vi "Prechirper response process.vi"(8 "error in (no error)":errorcluster, 10 "Prechirper response":string, 11 "Pre-chirper commands":T1) -> (0 "error out":errorcluster, 2 "offset past number":i32, 3 "number":dbl)   [LabVIEW 2020]
uses:
  Prechirper commands.ctl
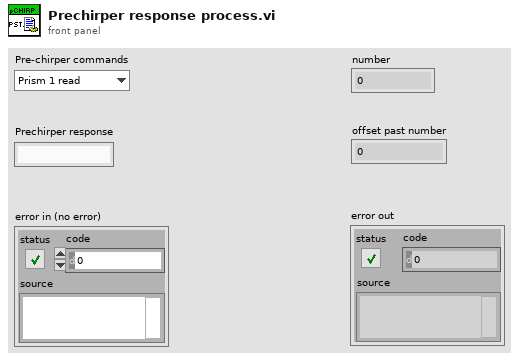
[diagram p1: front panel]
types:
  T1 = typedef "Prechirper commands.ctl" = enum16{"Prism 1 read", "Prism 1 set", "Prism 2 read", "Prism 2 set", "Wavelength read", "Wavelength Femto set", "Wavelength Femto and Laser set", "GVD curve number read", "GVD curve number set"}
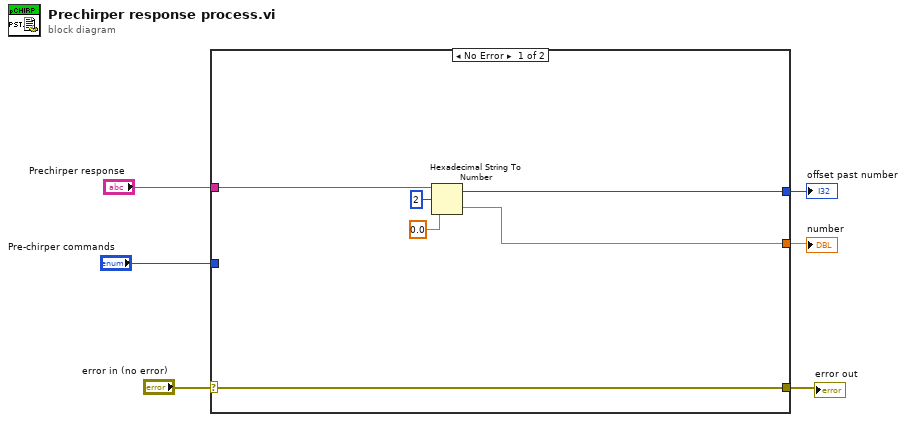
[diagram p0: block diagram]
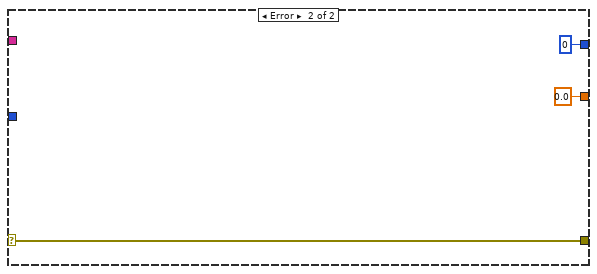
[diagram p2: hidden frame]
diagram:
  n1 = case shown="No Error" "error in (no error)" {
    selector: "error in (no error)" -> [w12 w13]
    tunnel: [w12 w13] -> w5
    tunnel: "Prechirper response" -> [w11 _]
    tunnel: "Pre-chirper commands" -> [_ _]
    tunnel: [w8 0.0] -> w2
    tunnel: [w7 0 ("offset past number")] -> w1
    frame No Error {
      n2 = Hexadecimal String To Number(string=w11, offset=2, default (0uL)=0.0) -> (offset past number=w7:i32, number=w8:dbl)
    }
    frame Error {
    }
  }
  "error out" <- w5
  "number" <- w2
  "offset past number" <- w1
